vi "Read Event Info.vi"(8 "error in (no error)":errorcluster, 11 "UserEventInfo in":refnum<class "UserEventInfo.lvclass">) -> (0 "error out":errorcluster, 2 "Event Info":T1, 3 "UserEventInfo out":refnum<class "UserEventInfo.lvclass">)   [LabVIEW 2019, in "EventRecorder.lvlib" / "UserEventInfo.lvclass"]
uses:
  UserEventInfo.lvclass
  UserEventInfo.lvclass/UserEventInfo.ctl
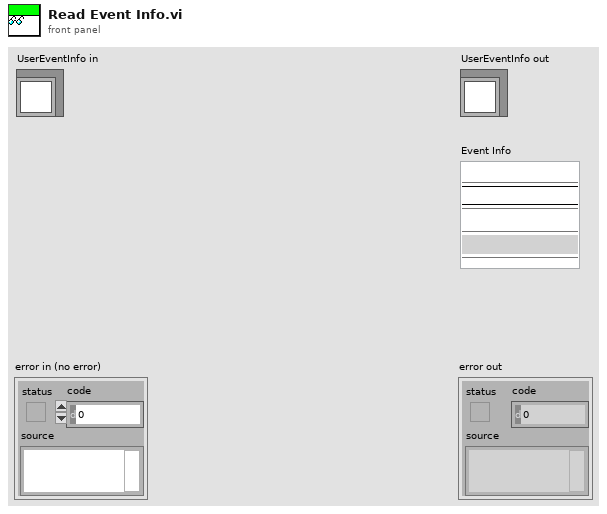
[diagram p1: front panel]
types:
  T1 = cluster{"Event Name":string, "Event Description":string}
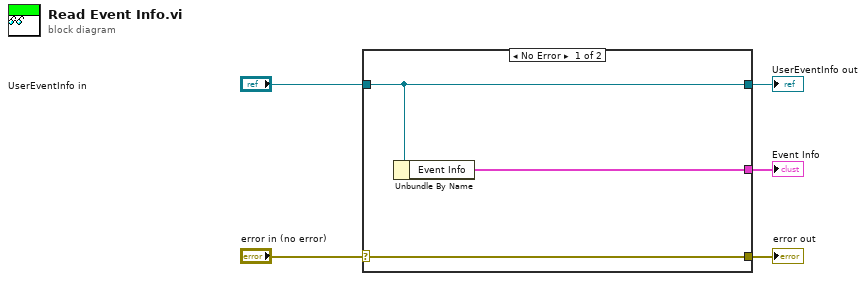
[diagram p0: block diagram]
diagram:
  n1 = case shown="No Error" "error in (no error)" {
    selector: "error in (no error)" -> [w8 w9]
    tunnel: [w8 w9] -> w4
    tunnel: [w7 w10] -> w2
    tunnel: "UserEventInfo in" -> [w7 w10]
    tunnel: [w6 _] -> w1
    frame No Error {
      n2 = Unbundle By Name(w7) -> ("Event Info"=w6:T1)
    }
    frame Error {
    }
  }
  "error out" <- w4
  "UserEventInfo out" <- w2
  "Event Info" <- w1
